vi "fgt set sensor Bypass Valve.vi"(8 "error in (no error)":errorcluster, 10 "open?":bool, 11 "sensorIndex":u32) -> (0 "error out":errorcluster)   [LabVIEW 2016, in "fgt_SDK.lvlib"]
doc: "Sets the state of the sensor's bypass valve. This feature is only available on NIFS devices."
uses:
  fgt_SDK.lvlib
  dlls/fgt_SDK_32.dll
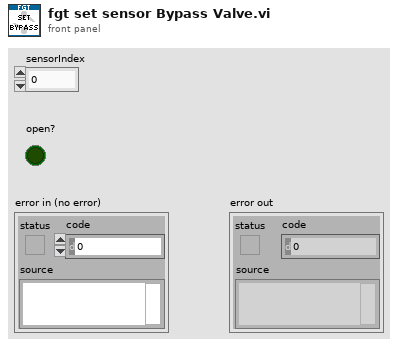
[diagram p1: front panel]
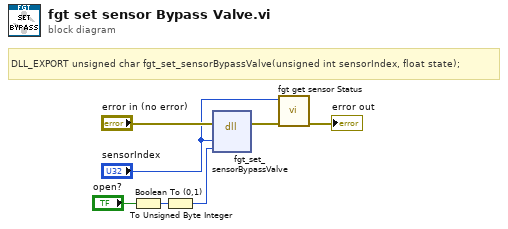
[diagram p0: block diagram]
diagram:
  # "DLL_EXPORT unsigned char fgt_set_sensorBypassValve(unsigned int sensorIndex, float state);"
  n1 = Boolean To (0,1)(Boolean="open?") -> (0, 1=w2:i16)
  n2 = To Unsigned Byte Integer(number=w2) -> (unsigned 8bit integer=w1:u8)
  n3 = dll-call lib="C:/projects/SDK/fgt-sdk-labview/dlls/fgt_SDK_*.*" fn="fgt_set_sensorBypassValve"(error in="error in (no error)", "sensorIndex"="sensorIndex", "value"=w1) -> (error out=w6:errorcluster)  [unwired: 5 in, 1 out]
  n4 = call "fgt get sensor Status.vi"("error in (no error)"=w6, "pressureIndex"="sensorIndex") -> ("error out"=→"error out":errorcluster)  [unwired: 9 in]
